vi "File RIO_Get Team Folder.vi"() -> (2 "error out":errorcluster, 3 "Team Files Folder":path)   [LabVIEW 2020]
panel:
  out "path":path
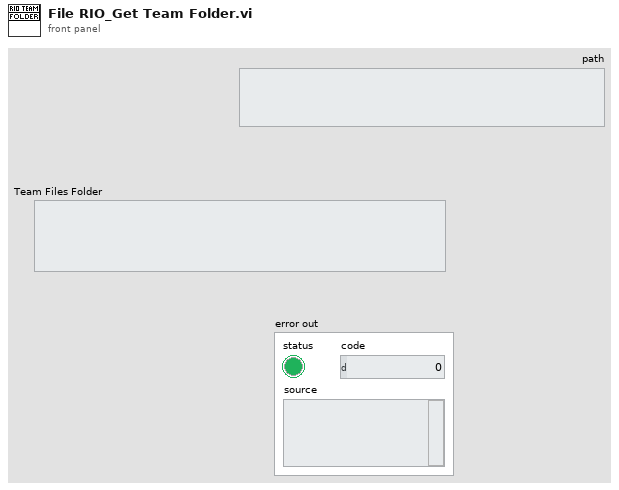
[diagram p1: front panel]
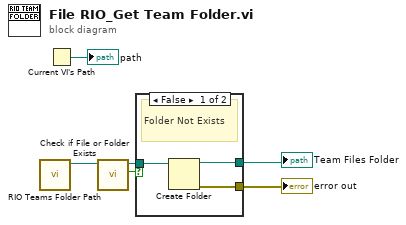
[diagram p0: block diagram]
diagram:
  n1 = call "RIO Teams Folder Path.vi"() -> ("Teams Folder"=w4:path)  [unwired: 10 in, 1 out]
  n2 = Current VI's Path() -> (path=→"path":path)
  n3 = call <vilib>:"Check if File or Folder Exists.vi"("path"=w4) -> ("file or folder exists?"=w2:bool, "dup path"=w3:path)  [unwired: 8 in, 1 out]
  n4 = case shown="False" w2 {
    tunnel: w3 -> [w9 w10]
    tunnel: [w8 _] -> w6
    tunnel: [w7 w10] -> w5
    frame False {
      # "Folder Not Exists"
      n5 = Create Folder(path (use dialog)=w9) -> (created path=w7:path, error out=w8:errorcluster)  [unwired: 2 in, 1 out]
    }
    frame True {
      # "Folder exists"
    }
  }
  "error out" <- w6
  "Team Files Folder" <- w5
